vi "COnfigure session.vi"(8 "error in (no error)":errorcluster, 9 "Tab control ref":refnum<vi>, 10 "password":string, 11 "username":string) -> (0 "error out":errorcluster, 3 "Session out":T1)   [LabVIEW 2020]
uses:
  <vilib>/httpClient/ClientHandle.ctl
  <vilib>/httpClient/LabVIEWHTTPClient.lvlib
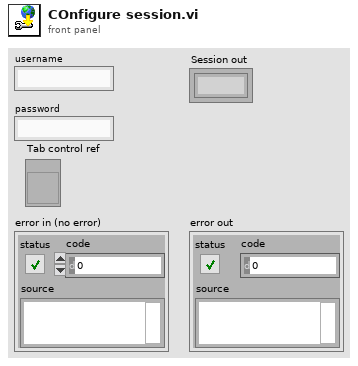
[diagram p1: front panel]
types:
  T1 = typedef "LabVIEWHTTPClient.lvlib/ClientHandle.ctl" = refnum<k1>
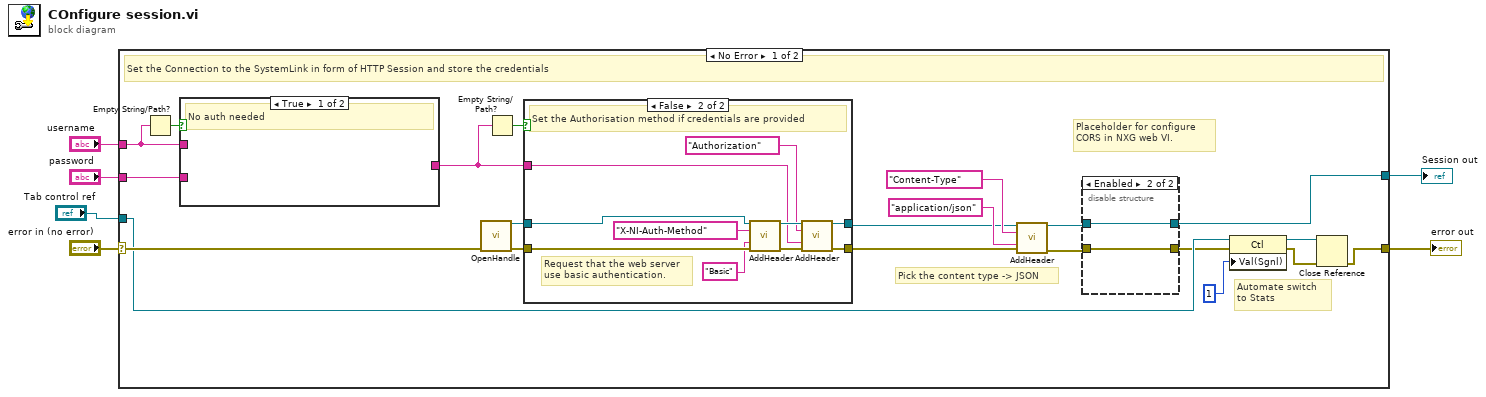
[diagram p0: block diagram]
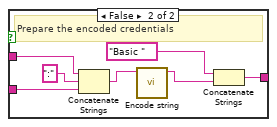
[diagram p3: hidden frame]
diagram:
  n1 = case shown="No Error" "error in (no error)" {
    selector: "error in (no error)" -> [w27 w51]
    tunnel: [w7 w51] -> w5
    tunnel: "password" -> [w26 _]
    tunnel: "username" -> [w25 _]
    tunnel: [w14 _] -> w2
    tunnel: "Tab control ref" -> [w11 _]
    frame No Error {
      # "Automate switch \nto Stats"
      # "Pick the content type -> JSON"
      # "Placeholder for configure CORS in NXG web VI."
      # "Set the Connection to the SystemLink in form of HTTP Session and store the credentials"
      n2 = Empty String/Path?(string/path=w25) -> (empty?=w23:bool)
      n3 = case shown="True" w23 {
        tunnel: w26 -> [_ w45]
        tunnel: w25 -> [_ w46]
        tunnel: [_ w42] -> w24
        frame True {
          # "No auth needed"
        }
        frame False {
          # "Prepare the encoded credentials"
          n4 = Concatenate Strings(w46, ":" ("string"), w45) -> (w41:string)
          n5 = call "Encode string.vi"("string"=w41) -> ("encoded string"=w40:string)  [unwired: 10 in]
          n6 = Concatenate Strings("Basic " ("string"), w40) -> (w42:string)
        }
      }
      n7 = call <vilib>:"OpenHandle.vi"("error in (no error)"=w27) -> ("client handle out"=w22:T1, "error out"=w21:errorcluster)  [unwired: 13 in]
      n8 = Empty String/Path?(string/path=w24) -> (empty?=w20:bool)
      n9 = case shown="False" w20 {
        tunnel: w21 -> [w29 w39]
        tunnel: [w29 w34] -> w17
        tunnel: w22 -> [w28 w37]
        tunnel: [w28 w32] -> w16
        tunnel: w24 -> [_ w30]
        frame True {
          # "No action"
        }
        frame False {
          # "Request that the web server use basic authentication."
          # "Set the Authorisation method if credentials are provided"
          n10 = call <vilib>:"AddHeader.vi"("client handle"=w37, "header"="X-NI-Auth-Method", "value"="Basic", "error in (no error)"=w39) -> ("client handle out"=w33:T1, "error out"=w38:errorcluster)  [unwired: 10 in]
          n11 = call <vilib>:"AddHeader.vi"("client handle"=w33, "header"="Authorization", "value"=w30, "error in (no error)"=w38) -> ("client handle out"=w32:T1, "error out"=w34:errorcluster)  [unwired: 10 in]
        }
      }
      n12 = call <vilib>:"AddHeader.vi"("client handle"=w16, "header"="Content-Type", "value"="application/json", "error in (no error)"=w17) -> ("client handle out"=w15:T1, "error out"=w13:errorcluster)  [unwired: 10 in]
      n13 = disable-structure shown="Enabled" {
        disable-tunnel: w13 -> [w48 w49]
        disable-tunnel: [w48 w49] -> w10
        disable-tunnel: w15 -> [w47 w50]
        disable-tunnel: [w47 w50] -> w14
        frame Disabled {
        }
        frame Enabled {
        }
      }
      n14 = property class="Ctl"(reference=w11, error in=w10, "Val(Sgnl)"=1) -> (reference out=w9:refnum<vi>, error out=w8:errorcluster)
      n15 = Close Reference(reference=w9, error in (no error)=w8) -> (error out=w7:errorcluster)
    }
    frame Error {
    }
  }
  "error out" <- w5
  "Session out" <- w2
